vi "test - Copy.vi"() -> ()   [LabVIEW 2025]
panel:
  in  "Number of trials":i32=1 min=1 step=1
  out "Final Door Probability":dbl
  out "Win Rate Stay":dbl
  out "Win Rate Switch":dbl
  in  "Number of Doors":dbl=3.0 min=3.0 step=1.0
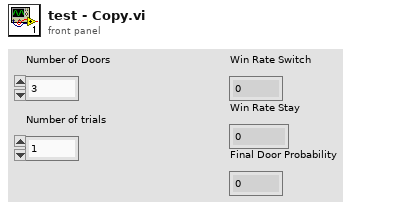
[diagram p1: front panel]
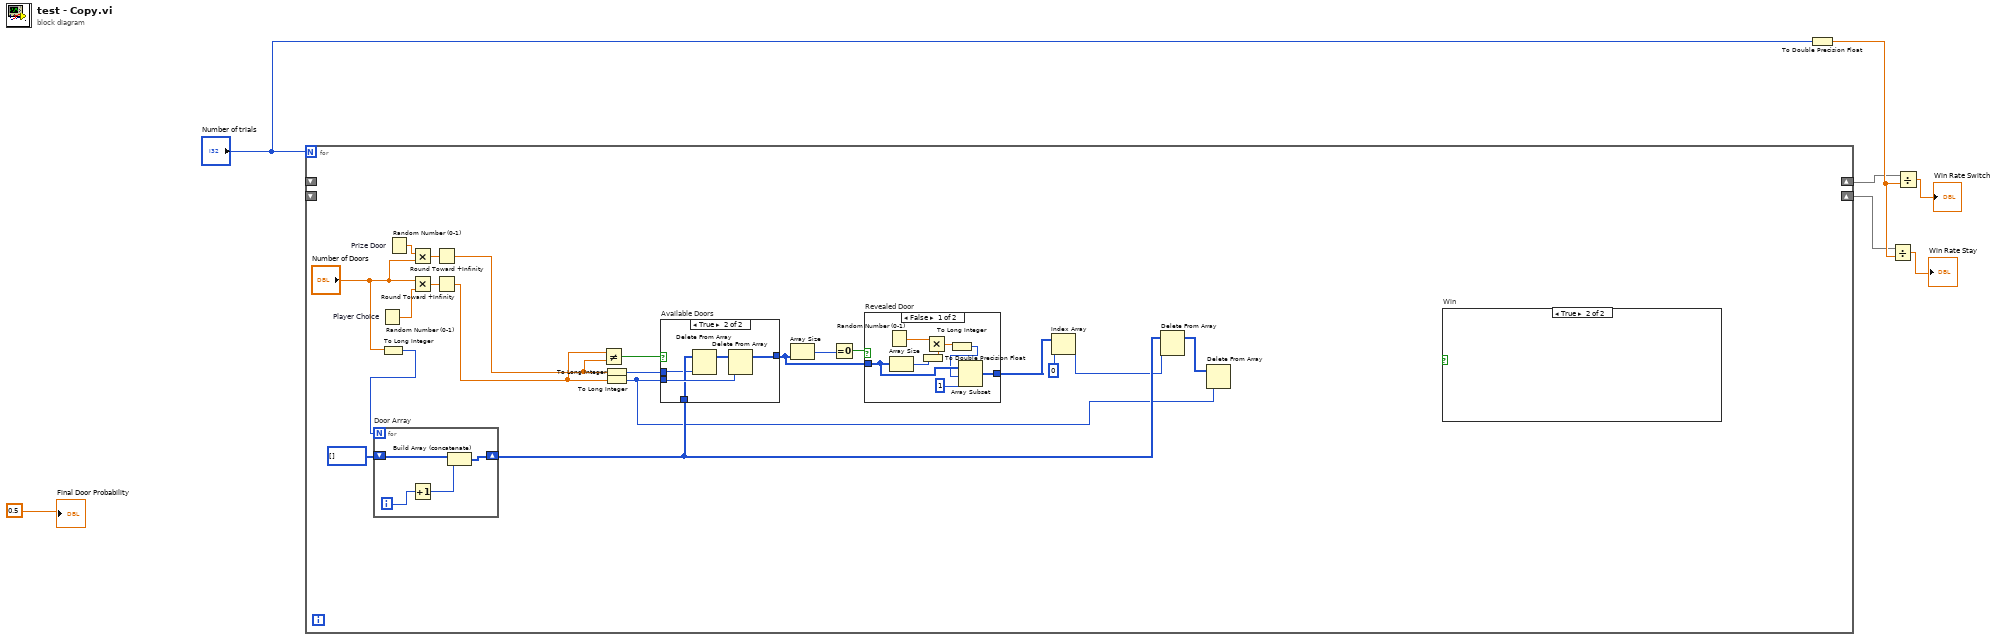
[diagram p0: block diagram]
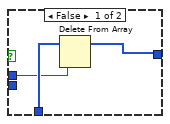
[diagram p4: hidden frame]
diagram:
  n1 = for {
    N: "Number of trials" -> [_]
    shift-right: [_] -> w4
    shift-left: _ -> [_]
    shift-right: [_] -> w3
    shift-left: _ -> [_]
    n2 = Random Number (0-1) "Player Choice"() -> (number: 0 to 1=w26:dbl)
    n3 = To Long Integer(number="Number of Doors") -> (32bit integer=w21:i32)
    n4 = for "Door Array" {
      N: w21 -> [_]
      shift-right: [w46] -> w11
      shift-left: i32[] [] -> [w45]
      i -> [w47]
      n5 = Increment(x=w47) -> (x+1=w44:i32)
      n6 = Build Array (concatenate)(w45, w44) -> (w46:i32[])
    }
    n7 = Random Number (0-1) "Prize Door"() -> (number: 0 to 1=w25:dbl)
    n8 = Multiply(x=w25, y="Number of Doors") -> (x*y=w24:dbl)
    n9 = Multiply(x="Number of Doors", y=w26) -> (x*y=w27:dbl)
    n10 = Round Toward +Infinity(x=w24) -> (ceil(x): smallest int >= x=w20:dbl)
    n11 = Round Toward +Infinity(x=w27) -> (ceil(x): smallest int >= x=w18:dbl)
    n12 = Not Equal?(x=w18, y=w20) -> (x != y?=w23:bool)
    n13 = To Long Integer(number=w20) -> (32bit integer=w19:i32)
    n14 = To Long Integer(number=w18) -> (32bit integer=w9:i32)
    n15 = case "Available Doors" shown="True" w23 {
      tunnel: w9 -> [_ w42]
      tunnel: w11 -> [w38 w41]
      tunnel: w19 -> [w37 w40]
      tunnel: [w36 w39] -> w15
      frame False {
        n16 = Delete From Array(array=w38, index=w37) -> (array with subset deleted=w36:i32[])  [unwired: 1 in, 1 out]
      }
      frame True {
        n17 = Delete From Array(array=w41, index=w40) -> (array with subset deleted=w43:i32[])  [unwired: 1 in, 1 out]
        n18 = Delete From Array(array=w43, index=w42) -> (array with subset deleted=w39:i32[])  [unwired: 1 in, 1 out]
      }
    }
    n19 = Array Size(array=w15) -> (size(s)=w16:i32)
    n20 = Equal To 0?(x=w16) -> (x = 0?=w14:bool)
    n21 = case "Revealed Door" shown="False" w14 {
      tunnel: w15 -> [w31 _]
      tunnel: [w28 _] -> w13
      frame False {
        n22 = Random Number (0-1)() -> (number: 0 to 1=w35:dbl)
        n23 = Array Size(array=w31) -> (size(s)=w34:i32)
        n24 = To Double Precision Float(number=w34) -> (double precision float=w33:dbl)
        n25 = Multiply(x=w35, y=w33) -> (x*y=w30:dbl)
        n26 = To Long Integer(number=w30) -> (32bit integer=w29:i32)
        n27 = Array Subset(array=w31, index=w29, length=1) -> (w28:i32[])
      }
      frame True {
      }
    }
    n28 = Index Array(array=w13, index=0) -> (element=w10:i32)
    n29 = Delete From Array "Delete From Array"(array=w11, index=w10) -> (array with subset deleted=w8:i32[])  [unwired: 1 in, 1 out]
    n30 = Delete From Array(array=w8, index=w9) -> ()  [unwired: 1 in, 2 out]
    n31 = case "Win" shown="True" {
      selector: _ -> [_ _]
      frame False {
      }
      frame True {
      }
    }
  }
  n32 = To Double Precision Float(number="Number of trials") -> (double precision float=w5:dbl)
  n33 = Divide(x=w3, y=w5) -> (x/y=→"Win Rate Stay":dbl)
  n34 = Divide(x=w4, y=w5) -> (x/y=→"Win Rate Switch":dbl)
  "Final Door Probability" <- 0.5
